vi "synth_subvi_rt.vi"(1 "A":dbl, 2 "fs [Hz]":dbl, 3 "fc [Hz]":dbl, 4 "time2":dbl[](array[numeric])=[0.0, 0.2, 0.25, 0.8, 1.0], 5 "w2(t)":dbl[](array[numeric])=[-40.0, 1.5, 0.0, 0.0, -40.0], 6 "time1":dbl[](array[numeric])=[0.0, 0.2, 0.25, 0.8, 1.0], 7 "w1(t)":dbl[](array[numeric])=[-40.0, 1.5, 0.0, 0.0, -40.0], 8 "duration [s]":dbl, 9 "H":dbl, 10 "Imin":dbl, 11 "Imax":dbl) -> (0 "discrete_sample":dbl[](array[numeric]))   [LabVIEW 2019]
uses:
  <vilib>/Analysis/1siggen.llb/Ramp Pattern by Samples.vi
  <vilib>/gmath/NI_Gmath.lvlib
  <vilib>/Analysis/NI_AALBase.lvlib
panel:
  out "Waveform":waveform(dbl)
  out "i(t)":dbl[](graph)
  out "a(t)":dbl[](graph)
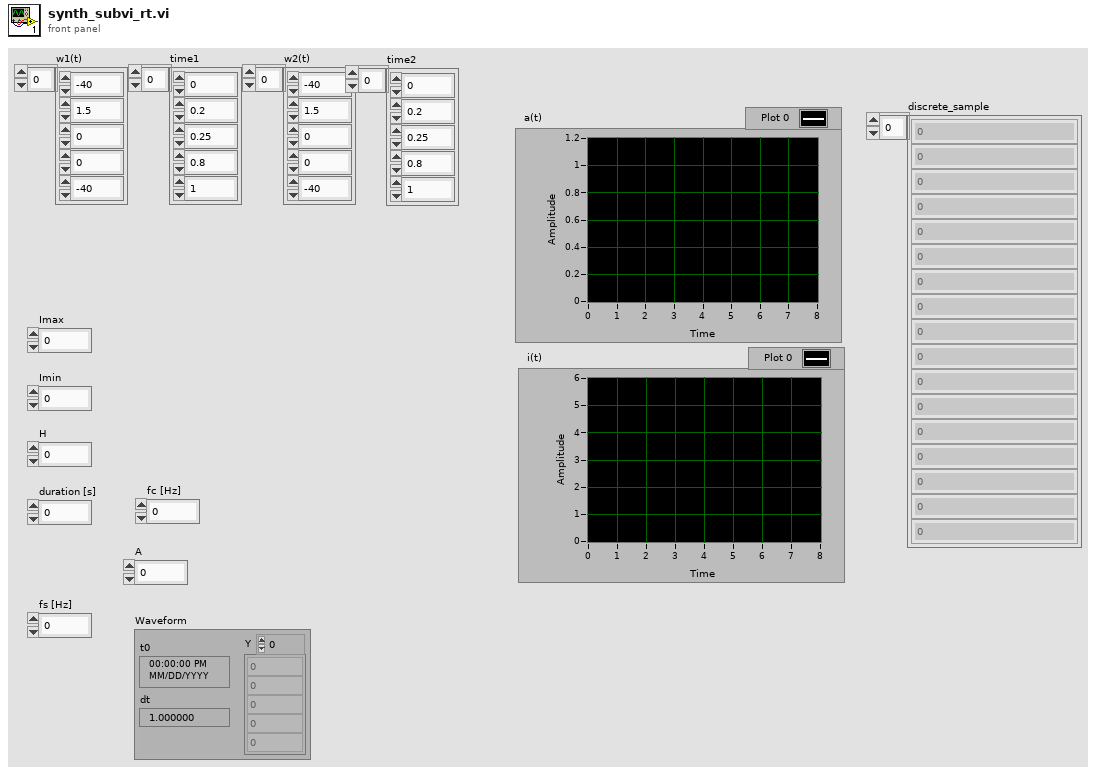
[diagram p1: front panel]
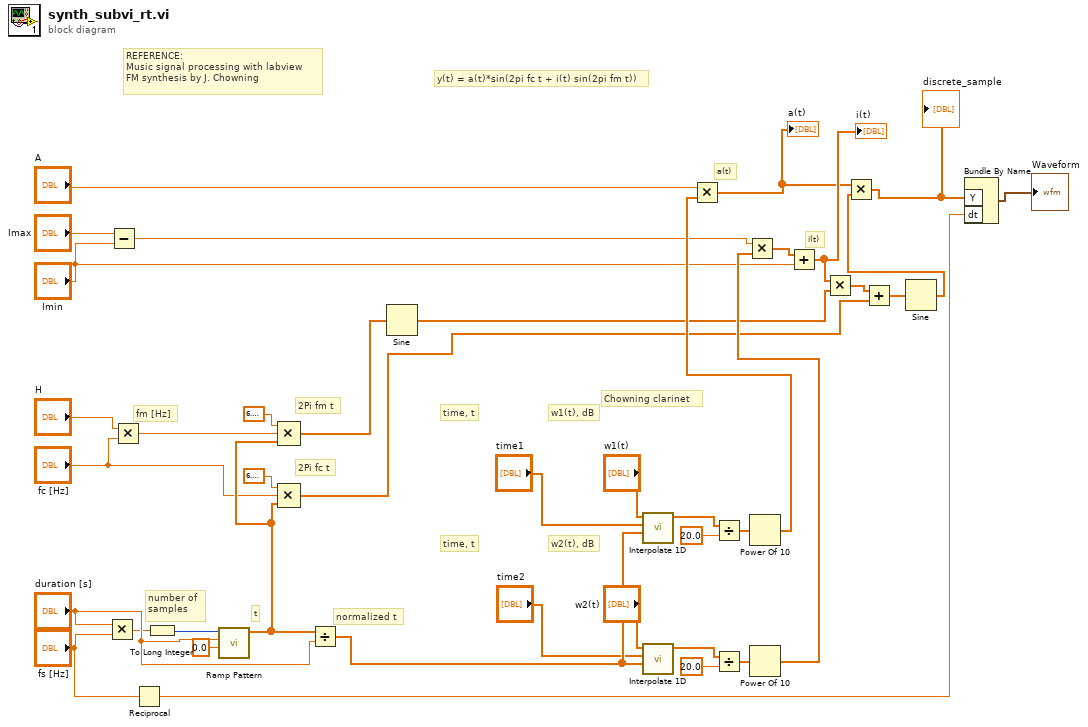
[diagram p0: block diagram]
diagram:
  # "y(t) = a(t)*sin(2pi fc t + i(t) sin(2pi fm t))"
  # "REFERENCE: \nMusic signal processing with labview\nFM synthesis by J. Chowning"
  # "i(t)"
  # "2Pi fm t"
  # "a(t)"
  # "w2(t), dB"
  # "time, t"
  # "normalized t"
  # "Chowning clarinet"
  # "w1(t), dB"
  # "time, t"
  # "fm [Hz]"
  # "2Pi fc t"
  # "t"
  # "number of\nsamples"
  n1 = Multiply(x="duration [s]", y="fs [Hz]") -> (x*y=w1:dbl)
  n2 = Subtract(x="Imax", y="Imin") -> (x-y=w24:dbl)
  n3 = Multiply(x="H", y="fc [Hz]") -> (x*y=w21:dbl)
  n4 = Reciprocal(x="fs [Hz]") -> (1/x=w35:dbl)
  n5 = To Long Integer(number=w1) -> (32bit integer=w2:i32)
  n6 = call-poly <vilib>:"Ramp Pattern.vi"("start"=0.0, "end"="duration [s]", "samples"=w2) -> ("Ramp Pattern"=w22:dbl[])  [unwired: 7 in, 1 out]
  n7 = Compound Arithmetic op=MULTIPLY(6.283185307179586, w21, w22) -> (w27:dbl[])
  n8 = Compound Arithmetic op=MULTIPLY(6.283185307179586, "fc [Hz]", w22) -> (w30:dbl[])
  n9 = Divide(x=w22, y="duration [s]") -> (x/y=w18:dbl[])
  n10 = Sine(x=w27) -> (sin(x)=w28:dbl[])
  n11 = call <vilib>:"Interpolate 1D.vi"("xi"=w18, "X"="time1", "Y"="w1(t)") -> ("yi"=w11:dbl[])  [unwired: 6 in, 2 out]
  n12 = call <vilib>:"Interpolate 1D.vi"("xi"=w18, "X"="time2", "Y"="w2(t)") -> ("yi"=w14:dbl[])  [unwired: 6 in, 2 out]
  n13 = Divide(x=w11, y=20.0) -> (x/y=w12:dbl[])
  n14 = Divide(x=w14, y=20.0) -> (x/y=w13:dbl[])
  n15 = Power Of 10(x=w12) -> (10^x=w31:dbl[])
  n16 = Multiply(x="A", y=w31) -> (x*y=w39:dbl[])
  "a(t)" <- w39
  n17 = Power Of 10(x=w13) -> (10^x=w32:dbl[])
  n18 = Multiply(x=w24, y=w32) -> (x*y=w25:dbl[])
  n19 = Add(x=w25, y="Imin") -> (x+y=w40:dbl[])
  "i(t)" <- w40
  n20 = Multiply(x=w40, y=w28) -> (x*y=w29:dbl[])
  n21 = Add(x=w29, y=w30) -> (x+y=w33:dbl[])
  n22 = Sine(x=w33) -> (sin(x)=w37:dbl[])
  n23 = Multiply(x=w39, y=w37) -> (x*y=w38:dbl[])
  "discrete_sample" <- w38
  n24 = Bundle By Name("Y"=w38, "dt"=w35) -> (→"Waveform":waveform(dbl))  [unwired: 1 in]
